vi "table size adjust (SubVI).vi"(10 "Array in":dbl[][](array[numeric]), 11 "xy cut pos correct":dbl[][](array[numeric])) -> (3 "Array out":dbl[][](array[numeric]))   [LabVIEW 2024]
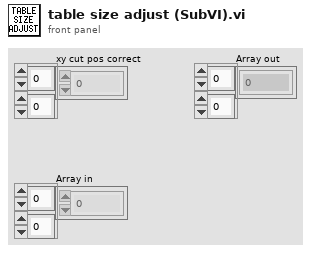
[diagram p1: front panel]
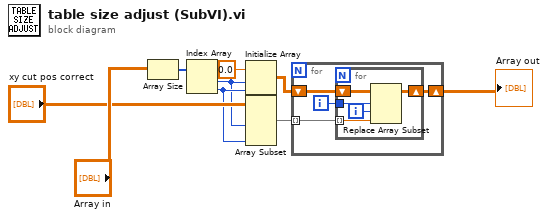
[diagram p0: block diagram]
diagram:
  n1 = Array Size(array="Array in") -> (size(s)=w1:i32[])
  n2 = Index Array(array=w1) -> (element #1=w3:i32, element #2=w4:i32)  [unwired: 2 in]
  n3 = Initialize Array(0.0 ("element"), w3, w4) -> (w6:dbl[][])
  n4 = Array Subset(array="xy cut pos correct", length (row)=w3, length (col)=w4) -> (w5:dbl[][])  [unwired: 2 in]
  n5 = for {
    tunnel: w5 -> [w13] mode=indexing
    shift-right: [w10] -> w8
    shift-left: w6 -> [w12]
    i -> [w11]
    n6 = for {
      tunnel: w13 -> [w15] mode=indexing
      tunnel: w11 -> [w16]
      shift-right: [w14] -> w10
      shift-left: w12 -> [w18]
      i -> [w17]
      n7 = Replace Array Subset(array=w18, new element=w15, index (row)=w16, index (col)=w17) -> (w14:dbl[][])
    }
  }
  "Array out" <- w8
